vi "Write concatenate pages dimensions.vi"(0 "PageSizeWithRotation":refnum<k24>, 5 "Pages [ ] IN":cluster{"Old":i32, "New":i32}[](array[cluster]), 7 "Pages dimensions [ ] IN original":T1[](array[typedef]) {"Page Size" items=["Custom", "LETTER", "NOTE", "LEGAL", "TABLOID", "EXECUTIVE", "POSTCARD", "A0", "A1", "A2", "A3", "A4", "A5", "A6", "A7", "A8", "A9", "A10", "B0", "B1", "B2", "B3", "B4", "B5", "B6", "B7", "B8", "B9", "B10", "ARCH_E", "ARCH_D", "ARCH_C", "ARCH_B", "ARCH_A", "FLSA", "FLSE", "HALFLETTER", "_11X17", "ID_1", "ID_2", "ID_3", "LEDGER", "CROWN_QUARTO", "LARGE_CROWN_QUARTO", "DEMY_QUARTO", "ROYAL_QUARTO", "CROWN_OCTAVO", "LARGE_CROWN_OCTAVO", "DEMY_OCTAVO", "ROYAL_OCTAVO", "SMALL_PAPERBACK", "PENGUIN_SMALL_PAPERBACK", "PENGUIN_LARGE_PAPERBACK"]}, 9 "Pages dimensions [ ] IN":T1[](array[typedef]) {"Page Size" items=["Custom", "LETTER", "NOTE", "LEGAL", "TABLOID", "EXECUTIVE", "POSTCARD", "A0", "A1", "A2", "A3", "A4", "A5", "A6", "A7", "A8", "A9", "A10", "B0", "B1", "B2", "B3", "B4", "B5", "B6", "B7", "B8", "B9", "B10", "ARCH_E", "ARCH_D", "ARCH_C", "ARCH_B", "ARCH_A", "FLSA", "FLSE", "HALFLETTER", "_11X17", "ID_1", "ID_2", "ID_3", "LEDGER", "CROWN_QUARTO", "LARGE_CROWN_QUARTO", "DEMY_QUARTO", "ROYAL_QUARTO", "CROWN_OCTAVO", "LARGE_CROWN_OCTAVO", "DEMY_OCTAVO", "ROYAL_OCTAVO", "SMALL_PAPERBACK", "PENGUIN_SMALL_PAPERBACK", "PENGUIN_LARGE_PAPERBACK"]}, 11 "error in (no error)":errorcluster, 12 "Old Page number":i32, 13 "PDF file source":T4, 14 "Actual Page number":i32) -> (4 "PageSizeWithRotation duplicate":refnum<k24>, 6 "Pages [ ] OUT":cluster{"Old":i32, "New":i32}[](array[cluster]), 10 "Pages dimensions OUT [ ]":T1[](array[typedef]) {"Page Size" items=["Custom", "LETTER", "NOTE", "LEGAL", "TABLOID", "EXECUTIVE", "POSTCARD", "A0", "A1", "A2", "A3", "A4", "A5", "A6", "A7", "A8", "A9", "A10", "B0", "B1", "B2", "B3", "B4", "B5", "B6", "B7", "B8", "B9", "B10", "ARCH_E", "ARCH_D", "ARCH_C", "ARCH_B", "ARCH_A", "FLSA", "FLSE", "HALFLETTER", "_11X17", "ID_1", "ID_2", "ID_3", "LEDGER", "CROWN_QUARTO", "LARGE_CROWN_QUARTO", "DEMY_QUARTO", "ROYAL_QUARTO", "CROWN_OCTAVO", "LARGE_CROWN_OCTAVO", "DEMY_OCTAVO", "ROYAL_OCTAVO", "SMALL_PAPERBACK", "PENGUIN_SMALL_PAPERBACK", "PENGUIN_LARGE_PAPERBACK"]}, 15 "error out":errorcluster)   [LabVIEW 2019]
doc: "Version 1.1\nDeveloped by Jean-Marc Simard\nCopyright © 2012, Exaprom Inc.\nAll rights reserved.\nLicense: BSD\n\nWith iTextSharp 4.1.6 (http://itextsharp.sourceforge.net)\nunder Mozilla Public License Version 1.1\n(http://www.mozilla.org/MPL/MPL-1.1.html)"
uses:
  <userlib>/Exaprom PDF/Controls/Page Controls/Page dimensions.ctl
  <userlib>/Exaprom PDF/Controls/Page Controls/Page size.ctl
  <userlib>/Exaprom PDF/Controls/Page Controls/Page Orientation.ctl
  C:/Program Files/National Instruments/LabVIEW 2019/user.lib/Exaprom PDF/DLL/itextsharp.dll
  DLL/itextsharp.dll
  <userlib>/Exaprom PDF/Controls/Concatenate Controls/PDF file source.ctl
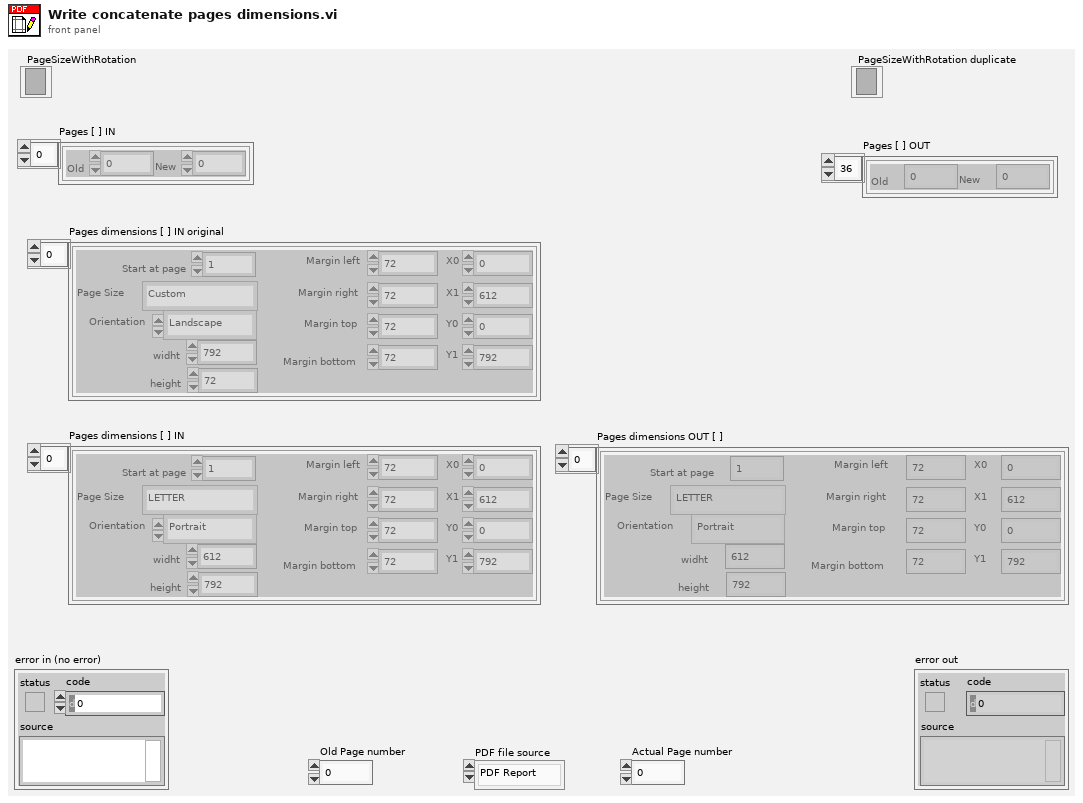
[diagram p1: front panel]
types:
  T1 = typedef "Page dimensions.ctl" = cluster{"Start at page":i32, "Page Size":T2, "Orientation":T3, "widht":sgl, "height":sgl, "Margin left":sgl, "Margin right":sgl, "Margin top":sgl, "Margin bottom":sgl, "X0":sgl, "X1":sgl, "Y0":sgl, "Y1":sgl}
  T2 = typedef "Page size.ctl" = i32
  T3 = typedef "Page Orientation.ctl" = enum16{"Portrait", "Landscape"}
  T4 = typedef "PDF file source.ctl" = enum16{"PDF Report", "File to add"}
  T5 = cluster{"Old Page number":i32, "Actual Page number":i32}
  T6 = cluster{"Old Page number":i32, "Actual Page number":i32}[]
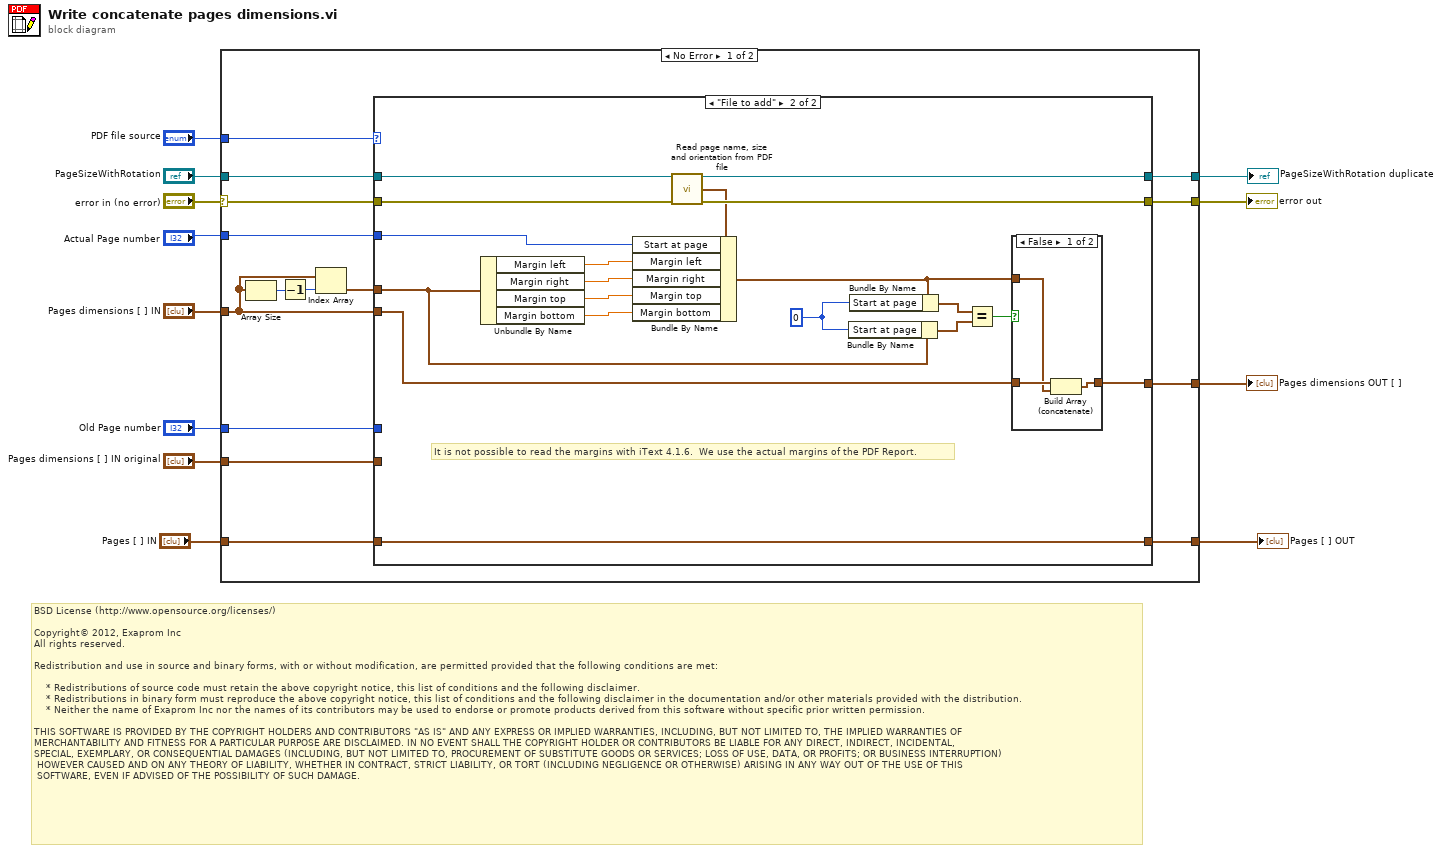
[diagram p0: block diagram]
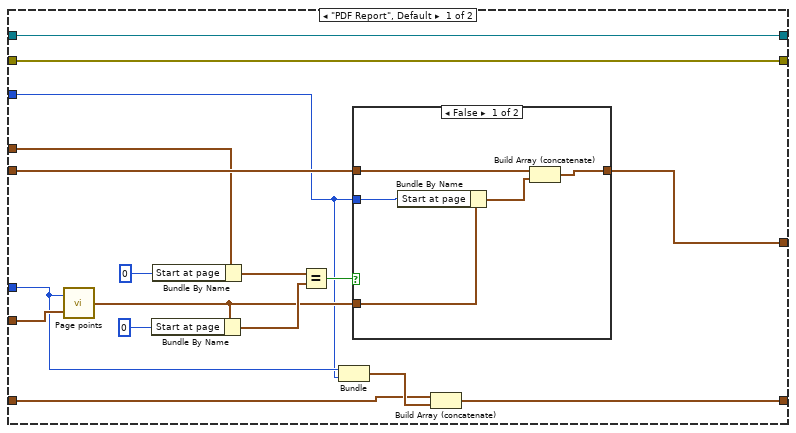
[diagram p2: hidden frame]
diagram:
  # "BSD License (http://www.opensource.org/licenses/)\n\nCopyright© 2012, Exaprom Inc\nAll rights reserved.\n\nRedistribution and use in source and binary forms, with or without modification, are permitted provided that the following conditions are met:\n\n    * Redistributions of source code must retain the above copyright notice, this list of conditions and the following disclaimer.\n    * Redistributions in binary form must reproduce the above copyright notice, this list of conditions and the following disclaimer in the documentation and/or other materials provided with the distribution.\n    * Neither the name of Exaprom Inc nor the names of its contributors may be used to endorse or promote products derived from this software without specific prior written permission.\n\nTHIS SOFTWARE IS PROVIDED BY THE COPYRIGHT HOLDERS AND CONTRIBUTORS \"AS IS\" AND ANY EXPRESS OR IMPLIED WARRANTIES, INCLUDING, BUT NOT LIMITED TO, THE IMPLIED WARRANTIES OF \nMERCHANTABILITY AND FITNESS FOR A PARTICULAR PURPOSE ARE DISCLAIMED. IN NO EVENT SHALL THE COPYRIGHT HOLDER OR CONTRIBUTORS BE LIABLE FOR ANY DIRECT, INDIRECT, INCIDENTAL,\nSPECIAL, EXEMPLARY, OR CONSEQUENTIAL DAMAGES (INCLUDING, BUT NOT LIMITED TO, PROCUREMENT OF SUBSTITUTE GOODS OR SERVICES; LOSS OF USE, DATA, OR PROFITS; OR BUSINESS INTERRUPTION)\n HOWEVER CAUSED AND ON ANY THEORY OF LIABILITY, WHETHER IN CONTRACT, STRICT LIABILITY, OR TORT (INCLUDING NEGLIGENCE OR OTHERWISE) ARISING IN ANY WAY OUT OF THE USE OF THIS\n SOFTWARE, EVEN IF ADVISED OF THE POSSIBILITY OF SUCH DAMAGE."
  n1 = case shown="No Error" "error in (no error)" {
    selector: "error in (no error)" -> [w23 w77]
    tunnel: [w25 w77] -> w12
    tunnel: "Actual Page number" -> [w22 _]
    tunnel: "Pages dimensions [ ] IN" -> [w16 w76]
    tunnel: [w27 w76] -> w8
    tunnel: "PageSizeWithRotation" -> [w24 w75]
    tunnel: [w26 w75] -> w6
    tunnel: "PDF file source" -> [w21 _]
    tunnel: "Old Page number" -> [w20 _]
    tunnel: "Pages dimensions [ ] IN original" -> [w19 _]
    tunnel: [w14 w74] -> w2
    tunnel: "Pages [ ] IN" -> [w13 w74]
    frame No Error {
      n2 = Array Size(array=w16) -> (size(s)=w17:i32)
      n3 = Decrement(x=w17) -> (x-1=w18:i32)
      n4 = Index Array(array=w16, index=w18) -> (element=w15:T1)
      n5 = case shown="\"File to add\"" w21 {
        tunnel: [w36 w60] -> w27
        tunnel: [w44 w59] -> w26
        tunnel: [w43 w58] -> w25
        tunnel: w24 -> [w44 w57]
        tunnel: w23 -> [w43 w56]
        tunnel: w22 -> [w31 w54]
        tunnel: w16 -> [w35 w53]
        tunnel: w20 -> [w32 _]
        tunnel: w19 -> [w42 _]
        tunnel: w15 -> [w33 w52]
        tunnel: [w29 w51] -> w14
        tunnel: w13 -> [w28 w51]
        frame "PDF Report", Default {
          n6 = call <userlib>:"Page points.vi"("Pages dimensions [ ]"=w42, "pageNum"=w32) -> ("Page (points)"=w34:T1)
          n7 = Bundle By Name(cluster=w34, "Start at page"=0) -> (w38:T1)
          n8 = Bundle By Name(cluster=w33, "Start at page"=0) -> (w39:T1)
          n9 = Equal?(x=w39, y=w38) -> (x = y?=w37:bool)
          n10 = Bundle("Old Page number"=w32, "Actual Page number"=w31) -> (w30:T5)  [unwired: 1 in]
          n11 = case shown="False" w37 {
            tunnel: [w48 w50] -> w36
            tunnel: w35 -> [w49 w50]
            tunnel: w34 -> [w45 _]
            tunnel: w31 -> [w47 _]
            frame False {
              n12 = Bundle By Name(cluster=w45, "Start at page"=w47) -> (w46:T1)
              n13 = Build Array (concatenate)(w49, w46) -> (w48:T1[])
            }
            frame True {
            }
          }
          n14 = Build Array (concatenate)(w28, w30) -> (w29:T6)
        }
        frame "File to add" {
          w65 = 0
          # "It is not possible to read the margins with iText 4.1.6.  We use the actual margins of the PDF Report."
          n15 = Unbundle By Name(w52) -> ("Margin left"=w69:sgl, "Margin right"=w68:sgl, "Margin top"=w67:sgl, "Margin bottom"=w66:sgl)
          n16 = call <userlib>:"Read page name, size and orientation from PDF file.vi"("PageSizeWithRotation"=w57, "error in (no error)"=w56) -> ("PageSizeWithRotation duplicate"=w59:refnum<k24>, "Pages dimensions OUT"=w55:T1, "error out"=w58:errorcluster)  [unwired: 11 in]
          n17 = Bundle By Name(cluster=w55, "Start at page"=w54, "Margin left"=w69, "Margin right"=w68, "Margin top"=w67, "Margin bottom"=w66) -> (w61:T1)
          n18 = Bundle By Name(cluster=w52, "Start at page"=w65) -> (w63:T1)
          n19 = Bundle By Name(cluster=w61, "Start at page"=w65) -> (w64:T1)
          n20 = Equal?(x=w64, y=w63) -> (x = y?=w62:bool)
          n21 = case shown="False" w62 {
            tunnel: w53 -> [w72 w73]
            tunnel: [w71 w73] -> w60
            tunnel: w61 -> [w70 _]
            frame False {
              n22 = Build Array (concatenate)(w72, w70) -> (w71:T1[])
            }
            frame True {
            }
          }
        }
      }
    }
    frame Error {
    }
  }
  "error out" <- w12
  "Pages dimensions OUT [ ]" <- w8
  "PageSizeWithRotation duplicate" <- w6
  "Pages [ ] OUT" <- w2
